vi "Connect.vi"(8 "error in (no error)":errorcluster, 10 "Connection list in":string, 11 "SLSC Switch Consumer in":refnum<class "SLSC Switch Consumer.lvclass">) -> (0 "error out":errorcluster, 3 "SLSC Switch Consumer out":refnum<class "SLSC Switch Consumer.lvclass">)   [LabVIEW 2017, in "SLSC Switch Messaging.lvlib" / "SLSC Switch Consumer.lvclass"]
uses:
  SLSC Switch Consumer.lvclass
  SLSC Switch Consumer.lvclass/SLSC Switch Consumer.ctl
  <vilib>/SLSC_Switch/Connect Channels (Multiple).vi
  <vilib>/SLSC_Switch/SLSC Switch.lvlib
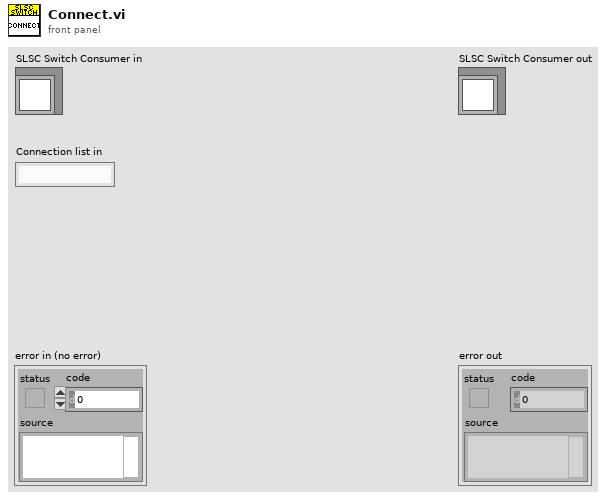
[diagram p1: front panel]
types:
  T1 = typedef "nislscslSession.ctl" = refnum<k20>
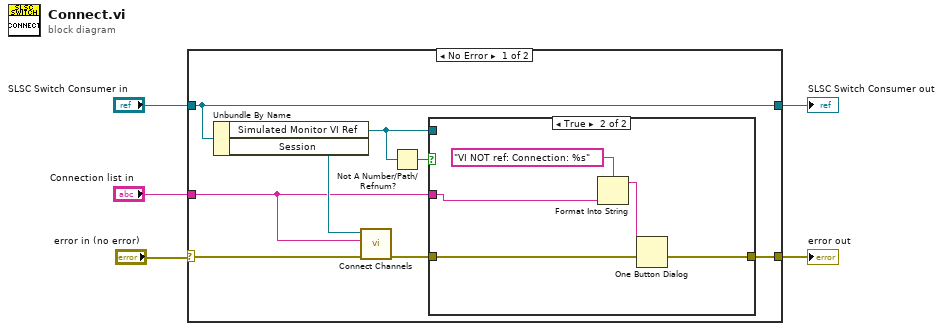
[diagram p0: block diagram]
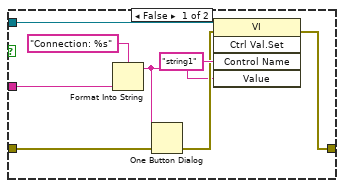
[diagram p2: hidden frame]
diagram:
  n1 = case shown="No Error" "error in (no error)" {
    selector: "error in (no error)" -> [w11 w26]
    tunnel: [w6 w26] -> w4
    tunnel: [w13 w25] -> w1
    tunnel: "SLSC Switch Consumer in" -> [w13 w25]
    tunnel: "Connection list in" -> [w8 _]
    frame No Error {
      n2 = Unbundle By Name(w13) -> ("Simulated Monitor VI Ref"=w10:refnum<vi>, "Session"=w12:T1)
      n3 = call-poly <vilib>:"Connect Channels.vi"("error in (no error)"=w11, "connection list"=w8, "session in"=w12) -> ("error out"=w7:errorcluster)  [unwired: 7 in, 1 out]
      n4 = Not A Number/Path/Refnum?(number/path/refnum=w10) -> (NaN/Path/Refnum?=w9:bool)
      n5 = case shown="True" w9 {
        tunnel: w10 -> [w19 _]
        tunnel: w8 -> [w17 w21]
        tunnel: w7 -> [w16 w24]
        tunnel: [w15 w24] -> w6
        frame False {
          n6 = Format Into String(format string="Connection: %s", w17) -> (resulting string=w14:string)  [unwired: 2 in, 1 out]
          n7 = One Button Dialog(message=w14) -> ()  [unwired: 1 in, 1 out]
          n8 = invoke class="VI" method="Ctrl Val.Set"(reference=w19, error in=w16, "Control Name"="string1", "Value"=w14) -> (error out=w15:errorcluster)  [unwired: 1 in, 4 out]
        }
        frame True {
          n9 = Format Into String(format string="VI NOT ref: Connection: %s", w21) -> (resulting string=w23:string)  [unwired: 2 in, 1 out]
          n10 = One Button Dialog(message=w23) -> ()  [unwired: 1 in, 1 out]
        }
      }
    }
    frame Error {
    }
  }
  "error out" <- w4
  "SLSC Switch Consumer out" <- w1
